vi "top line of segmented image.vi"(11 "Array":sgl[](array[numeric])) -> (3 "Numeric":i32)   [LabVIEW 2011]
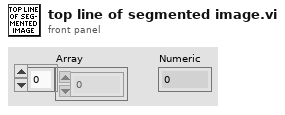
[diagram p1: front panel]
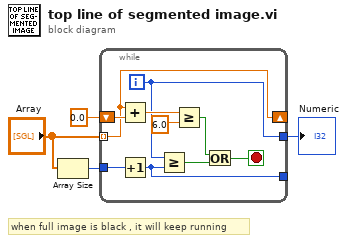
[diagram p0: block diagram]
diagram:
  # "when full image is black , it will keep running"
  n1 = Array Size(array="Array") -> (size(s)=w1:i32)
  n2 = while {
    tunnel: "Array" -> [w13] mode=indexing
    shift-right: [w13] -> _
    shift-left: sgl 0.0 -> [w14]
    tunnel: [w10] -> w4
    tunnel: [w5] -> _
    tunnel: w1 -> [w9]
    i -> [w10]
    stop <- w6 stop-if-true
    n3 = Add(x=w13, y=w14) -> (x+y=w12:sgl)
    n4 = Increment(x=w9) -> (x+1=w5:i32)
    n5 = Greater Or Equal?(x=w10, y=w5) -> (x >= y?=w8:bool)
    n6 = Greater Or Equal?(x=w12, y=sgl 6.0) -> (x >= y?=w7:bool)
    n7 = Or(x=w7, y=w8) -> (x .or. y?=w6:bool)
  }
  "Numeric" <- w4
